vi "Solve_Special_PRB_101_Subtracks-3.vi"(3 "error IN":errorcluster, 5 "[IN] Subtracks":T1(array[cluster])) -> (0 "error OUT":errorcluster, 1 "[OUT] Special case!":bool, 2 "[OUT] Subtracks":T1(array[cluster]))   [LabVIEW 2013]
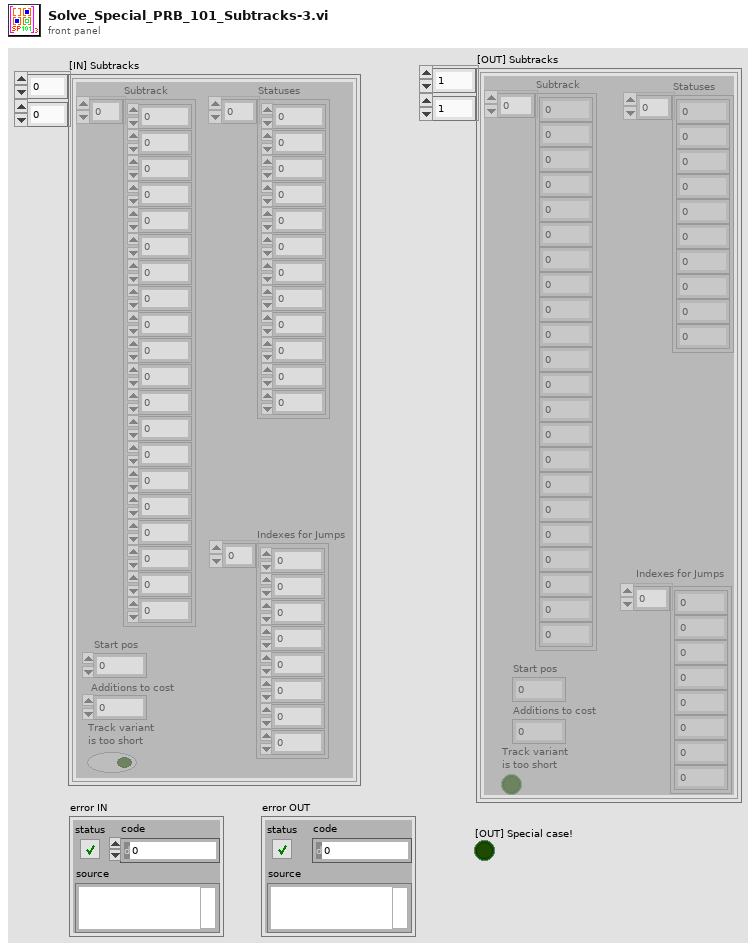
[diagram p1: front panel]
types:
  T1 = cluster{"Subtrack":dbl[], "Statuses":i16[], "Start pos":i32, "Additions to cost":i32, "Track variant \nis too short":bool, "Indexes for Jumps":i32[]}[][]
  T2 = cluster{"Subtrack":dbl[], "Statuses":i16[], "Start pos":i32, "Additions to cost":i32, "Track variant \nis too short":bool, "Indexes for Jumps":i32[]}
  T3 = cluster{"Subtrack":dbl[], "Statuses":i16[], "Start pos":i32, "Additions to cost":i32, "Track variant \nis too short":bool, "Indexes for Jumps":i32[]}[]
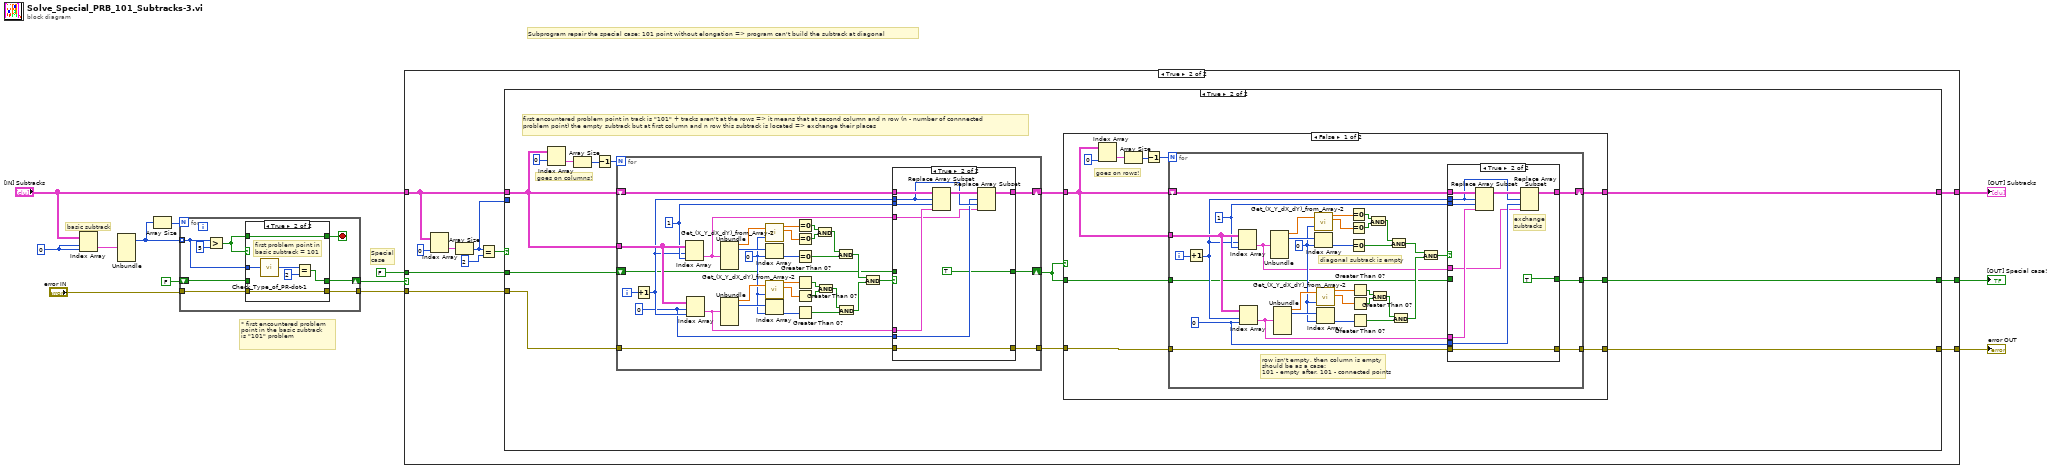
[diagram p0: block diagram]
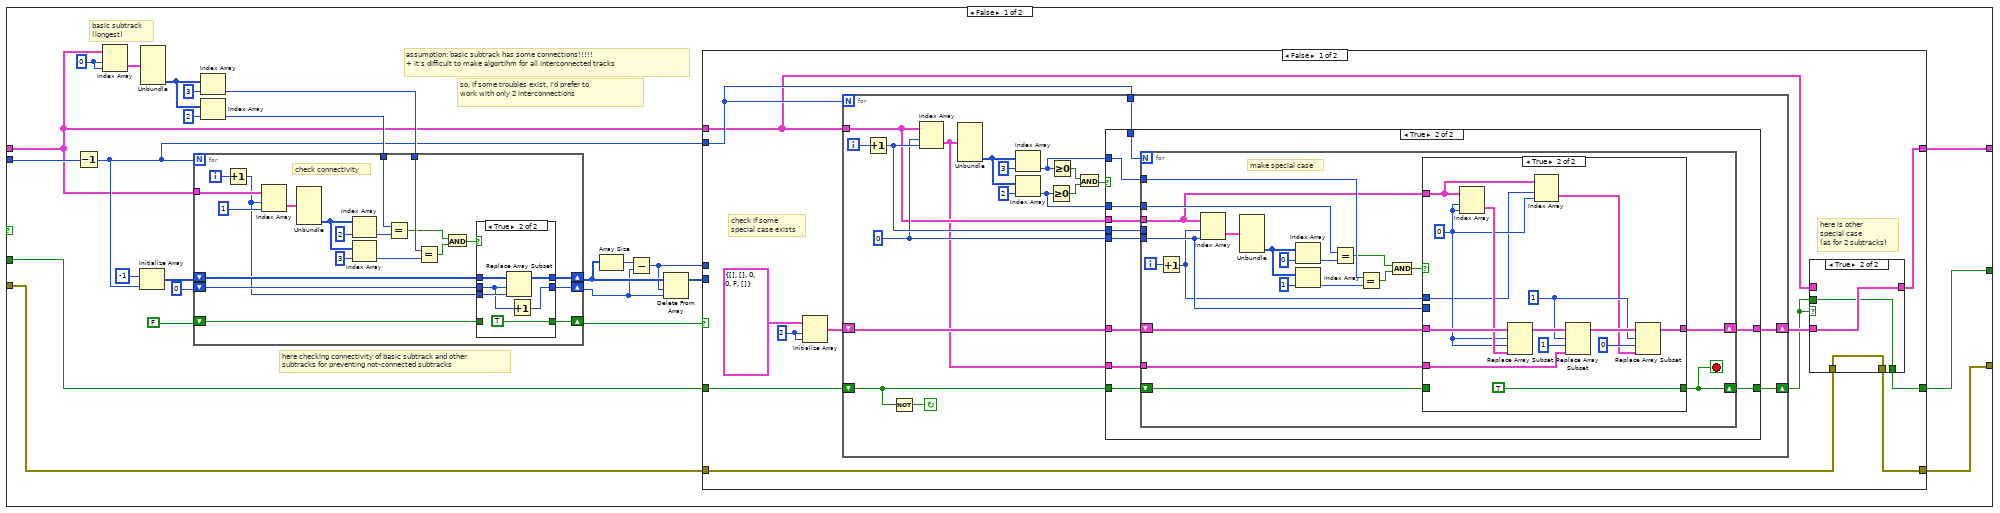
[diagram p3: hidden frame]
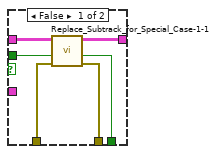
[diagram p4: hidden frame]
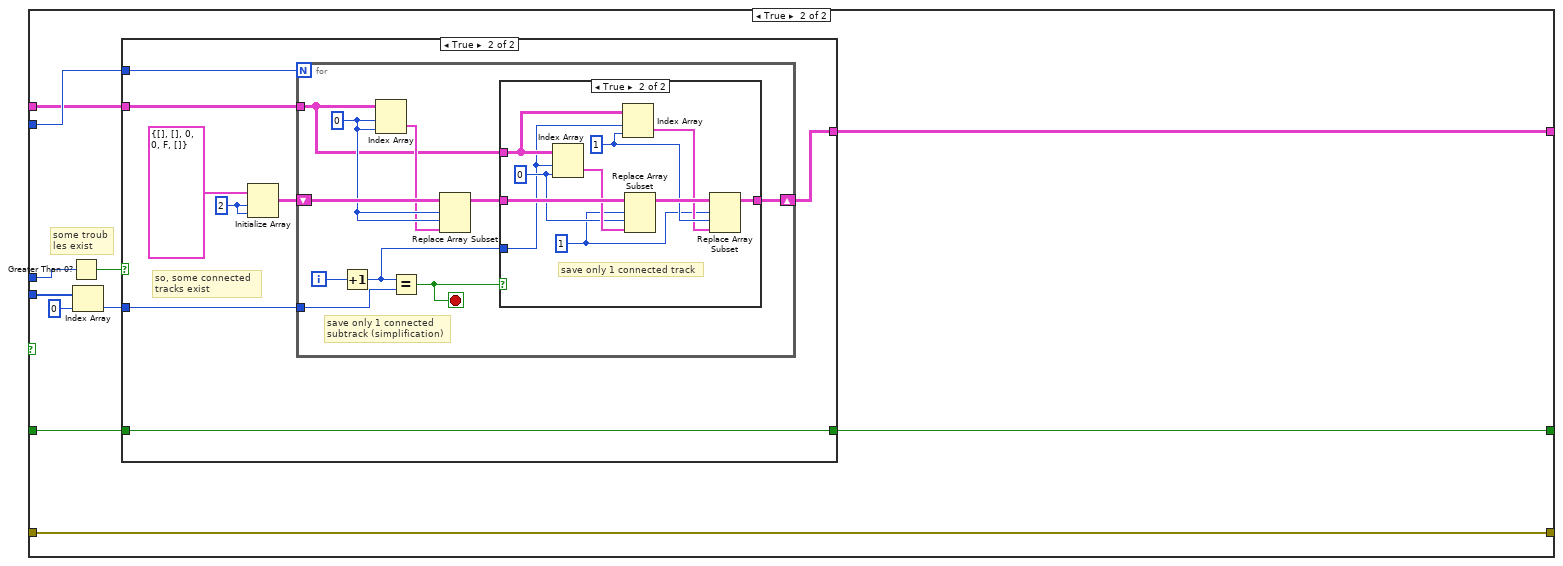
[diagram p7: hidden frame]
diagram:
  w13 = 0 ("index (row)")
  # "* first encountered problem\npoint in the basic subtrack\nis \"101\" problem"
  # "Special \ncase"
  # "Subprogram repair the special case: 101 point without elongation => program can't build the subtrack at diagonal"
  # "basic subtrack"
  n1 = Index Array(array="[IN] Subtracks", index (row)=w13, index (col)=w13) -> (element=w12:T2)
  n2 = Unbundle(w12) -> ("Statuses"=w10:i16[])  [unwired: 5 out]
  n3 = Array Size(array=w10) -> (size(s)=w11:i32)
  n4 = for {
    N: w11 -> [_]
    tunnel: w10 -> [w20] mode=indexing
    shift-right: [w16] -> w1
    shift-left: FALSE -> [w19]
    tunnel: "error IN" -> [w15]
    tunnel: [w14] -> w7
    stop <- w17 stop-if-true
    n5 = Greater?(x=w20, y=i16 5) -> (0:w18:bool)
    n6 = case shown="True" w18 {
      tunnel: w20 -> [_ w28]
      tunnel: w19 -> [w23 _]
      tunnel: w18 -> [w24 w27]
      tunnel: [w24 w27] -> w17
      tunnel: [w23 w26] -> w16
      tunnel: w15 -> [w22 w25]
      tunnel: [w22 w25] -> w14
      frame False {
      }
      frame True {
        # "first problem point in \nbasic subtrack = 101"
        n7 = call "Check_Type_of_PR-dot-1.vi"("[IN] dot status"=w28) -> ("[OUT] Type of\nproblem dot"=w30:i32)
        n8 = Equal?(x=w30, y=2) -> (x = y?=w26:bool)
      }
    }
  }
  n9 = case shown="True" w1 {
    tunnel: w7 -> [w31 w44]
    tunnel: "[IN] Subtracks" -> [w33 w39]
    tunnel: FALSE -> [w32 w43]
    tunnel: [w32 w42] -> w4
    tunnel: [w33 w41] -> w3
    tunnel: [w31 w40] -> w2
    frame False {
    }
    frame True {
      n10 = Index Array(array=w39, index (col)=0) -> (element=w37:T3)  [unwired: 1 in]
      n11 = Array Size(array=w37) -> (size(s)=w34:i32)
      n12 = Equal?(x=w34, y=2) -> (x = y?=w35:bool)
      n13 = case shown="True" w35 {
        tunnel: w44 -> [w48 w243]
        tunnel: w39 -> [w50 w242]
        tunnel: w43 -> [w68 w241]
        tunnel: [w46 w237] -> w42
        tunnel: [w45 w236] -> w41
        tunnel: [w47 w235] -> w40
        tunnel: w34 -> [w69 _]
        frame False {
          w67 = 0 ("index (row)")
          # "so, if some troubles exist, I'd prefer to \nwork with only 2 interconnections"
          # "assumption: basic subtrack has some connections!!!!!\n+ it's difficult to make algortihm for all interconnected tracks"
          # "here checking connectivity of basic subtrack and other \nsubtracks for preventing not-connected subtracks"
          # "basic subtrack \n(longest)"
          n14 = Decrement(x=w69) -> (x-1=w52:i32)
          n15 = Index Array(array=w50, index (row)=w67, index (col)=w67) -> (element=w66:T2)
          n16 = Initialize Array(-1, w52) -> (w59:i32[])
          n17 = Unbundle(w66) -> ("Indexes for Jumps"=w63:i32[])  [unwired: 5 out]
          n18 = Index Array(array=w63, index=3) -> (element=w60:i32)
          n19 = Index Array(array=w63, index=2) -> (element=w61:i32)
          n20 = for {
            N: w52 -> [_]
            tunnel: w61 -> [w213]
            tunnel: w60 -> [w211]
            shift-right: [w204] -> w56
            shift-left: w59 -> [w207]
            shift-right: [w201] -> w51
            shift-left: FALSE -> [w203]
            shift-right: [w202] -> w54
            shift-left: 0 -> [w206]
            tunnel: w50 -> [w221]
            i -> [w220]
            # "check connectivity"
            n21 = Increment(x=w220) -> (x+1=w205:i32)
            n22 = Index Array(array=w221, index (row)=w205, index (col)=1) -> (element=w216:T2)
            n23 = Unbundle(w216) -> ("Indexes for Jumps"=w215:i32[])  [unwired: 5 out]
            n24 = Index Array(array=w215, index=2) -> (element=w214:i32)
            n25 = Index Array(array=w215, index=3) -> (element=w212:i32)
            n26 = Equal?(x=w213, y=w214) -> (x = y?=w210:bool)
            n27 = Equal?(x=w211, y=w212) -> (x = y?=w209:bool)
            n28 = And(x=w210, y=w209) -> (x .and. y?=w208:bool)
            n29 = case shown="True" w208 {
              tunnel: w207 -> [w222 w230]
              tunnel: w206 -> [w223 w227]
              tunnel: w205 -> [_ w229]
              tunnel: [w222 w228] -> w204
              tunnel: w203 -> [w224 _]
              tunnel: [w223 w226] -> w202
              tunnel: [w224 TRUE] -> w201
              frame False {
              }
              frame True {
                n30 = Replace Array Subset(array=w230, new element=w229, index=w227) -> (w228:i32[])
                n31 = Increment(x=w227) -> (x+1=w226:i32)
              }
            }
          }
          n32 = Array Size(array=w56) -> (size(s)=w55:i32)
          n33 = Subtract(x=w55, y=w54) -> (x-y=w49:i32)
          n34 = Delete From Array(array=w56, length=w49, index=w54) -> (array with subset deleted=w53:i32[])  [unwired: 1 out]
          n35 = case shown="False" w51 {
            tunnel: w53 -> [_ w165]
            tunnel: w52 -> [w80 w169]
            tunnel: w50 -> [w74 w168]
            tunnel: w68 -> [w81 w162]
            tunnel: w49 -> [_ w167]
            tunnel: w48 -> [w73 w159]
            tunnel: [w72 w159] -> w47
            tunnel: [w75 w161] -> w45
            tunnel: [w70 w160] -> w46
            frame False {
              w78 = 2 ("dimension size")
              # "here is other \nspecial case\n(as for 2 subtracks)"
              # "check if some \nspecial case exists"
              n36 = Initialize Array(T2 {"Subtrack"=[], "Statuses"=[], "Start pos"=0, "Additions to cost"=0, "Track variant \nis too short"=FALSE, "Indexes for Jumps"=[]} ("element"), w78, w78) -> (w77:T1)
              n37 = for {
                N: w80 -> [_]
                shift-right: [w98] -> w71
                shift-left: w81 -> [w95]
                tunnel: w80 -> [w99]
                tunnel: w74 -> [w97]
                shift-right: [w94] -> w76
                shift-left: w77 -> [w96]
                i -> [w109]
                stop <- w93 continue-if-true
                w102 = 0 ("disabled index (col)")
                n38 = Increment(x=w109) -> (x+1=w103:i32)
                n39 = Not(x=w95) -> (.not. x?=w93:bool)
                n40 = Index Array(array=w97, index (row)=w102, index (col)=w103) -> (element=w91:T2)
                n41 = Unbundle(w91) -> ("Indexes for Jumps"=w106:i32[])  [unwired: 5 out]
                n42 = Index Array(array=w106, index=3) -> (element=w100:i32)
                n43 = Index Array(array=w106, index=2) -> (element=w101:i32)
                n44 = Greater Or Equal To 0?(x=w101) -> (x >= 0?=w104:bool)
                n45 = Greater Or Equal To 0?(x=w100) -> (x >= 0?=w105:bool)
                n46 = And(x=w105, y=w104) -> (x .and. y?=w92:bool)
                n47 = case shown="True" w92 {
                  tunnel: w97 -> [_ w122]
                  tunnel: w103 -> [_ w121]
                  tunnel: w102 -> [_ w120]
                  tunnel: w101 -> [_ w119]
                  tunnel: w100 -> [_ w118]
                  tunnel: w99 -> [_ w117]
                  tunnel: w95 -> [w110 w116]
                  tunnel: [w110 w115] -> w98
                  tunnel: w96 -> [w111 w114]
                  tunnel: [w111 w113] -> w94
                  tunnel: w91 -> [_ w112]
                  frame False {
                  }
                  frame True {
                    n48 = for {
                      N: w117 -> [_]
                      tunnel: w121 -> [_]
                      tunnel: w120 -> [w132]
                      tunnel: w119 -> [w138]
                      tunnel: w118 -> [w137]
                      shift-right: [w126] -> w115
                      shift-left: w116 -> [w131]
                      tunnel: w122 -> [w133]
                      shift-right: [w127] -> w113
                      shift-left: w114 -> [w129]
                      tunnel: w112 -> [w123]
                      i -> [w125]
                      stop <- w126 stop-if-true
                      # "make special case"
                      n49 = Increment(x=w125) -> (x+1=w124:i32)
                      n50 = Index Array(array=w133, index (row)=w124, index (col)=w132) -> (element=w128:T2)
                      n51 = Unbundle(w128) -> ("Indexes for Jumps"=w140:i32[])  [unwired: 5 out]
                      n52 = Index Array(array=w140, index=0) -> (element=w139:i32)
                      n53 = Index Array(array=w140, index=1) -> (element=w136:i32)
                      n54 = Equal?(x=w138, y=w139) -> (x = y?=w135:bool)
                      n55 = Equal?(x=w137, y=w136) -> (x = y?=w134:bool)
                      n56 = And(x=w135, y=w134) -> (x .and. y?=w130:bool)
                      n57 = case shown="True" w130 {
                        tunnel: w133 -> [_ w148]
                        tunnel: w124 -> [_ w147]
                        tunnel: w132 -> [_ _]
                        tunnel: w131 -> [w144 _]
                        tunnel: [w144 TRUE] -> w126
                        tunnel: w129 -> [w143 w157]
                        tunnel: w123 -> [_ w153]
                        tunnel: [w143 w150] -> w127
                        frame False {
                        }
                        frame True {
                          w146 = 1 ("disabled index (col)")
                          w149 = 0 ("index (row)")
                          n58 = Index Array(array=w148, index (row)=w149, index (col)=w149) -> (element=w156:T2)
                          n59 = Replace Array Subset(array=w157, new element=w156, index (row)=w149, index (col)=w149) -> (w155:T1)
                          n60 = Index Array(array=w148, index (row)=w147, index (col)=w149) -> (element=w145:T2)
                          n61 = Replace Array Subset(array=w155, new element=w153, index (row)=w146, index (col)=1 ("disabled index (col)")) -> (w152:T1)
                          n62 = Replace Array Subset(array=w152, new element=w145, index (row)=w146, index (col)=0 ("disabled index (col)")) -> (w150:T1)
                        }
                      }
                    }
                  }
                }
              }
              n63 = case shown="True" w71 {
                tunnel: w76 -> [_ w90]
                tunnel: [w82 w90] -> w75
                tunnel: w74 -> [w87 _]
                tunnel: w73 -> [w86 w89]
                tunnel: [w85 w89] -> w72
                tunnel: w71 -> [w84 w88]
                tunnel: [w83 w88] -> w70
                frame False {
                  n64 = call "Replace_Subtrack_for_Special_Case-1-1.vi"("error IN"=w86, "[IN] Special case?"=w84, "[IN] Subtracks"=w87) -> ("error OUT"=w85:errorcluster, "[OUT Special case?"=w83:bool, "[OUT] Subtracks"=w82:T1)  [unwired: 2 in]
                }
                frame True {
                }
              }
            }
            frame True {
              # "some troub\nles exist"
              n65 = Greater Than 0?(x=w167) -> (x > 0?=w166:bool)
              n66 = Index Array(array=w165, index=0) -> (element=w163:i32)
              n67 = case shown="True" w166 {
                tunnel: w169 -> [_ w179]
                tunnel: w168 -> [w171 w177]
                tunnel: w163 -> [_ w178]
                tunnel: w162 -> [w170 w173]
                tunnel: [w170 w173] -> w160
                tunnel: [w171 w172] -> w161
                frame False {
                  # "no troubles => save all subtracks"
                }
                frame True {
                  w175 = 2 ("dimension size")
                  # "so, some connected \ntracks exist"
                  n68 = Initialize Array(T2 {"Subtrack"=[], "Statuses"=[], "Start pos"=0, "Additions to cost"=0, "Track variant \nis too short"=FALSE, "Indexes for Jumps"=[]} ("element"), w175, w175) -> (w174:T1)
                  n69 = for {
                    N: w179 -> [_]
                    tunnel: w178 -> [w188]
                    tunnel: w177 -> [w182]
                    shift-right: [w181] -> w172
                    shift-left: w174 -> [w187]
                    i -> [w189]
                    stop <- w183 stop-if-true
                    w186 = 0 ("index (row)")
                    # "save only 1 connected \nsubtrack (simplification)"
                    n70 = Increment(x=w189) -> (x+1=w180:i32)
                    n71 = Index Array(array=w182, index (row)=w186, index (col)=w186) -> (element=w185:T2)
                    n72 = Equal?(x=w180, y=w188) -> (x = y?=w183:bool)
                    n73 = Replace Array Subset(array=w187, new element=w185, index (row)=w186, index (col)=w186) -> (w184:T1)
                    n74 = case shown="True" w183 {
                      tunnel: w184 -> [w190 w200]
                      tunnel: w182 -> [_ w197]
                      tunnel: [w190 w192] -> w181
                      tunnel: w180 -> [_ w195]
                      frame False {
                      }
                      frame True {
                        w191 = 1 ("disabled index (row)")
                        w194 = 1 ("disabled index (col)")
                        w198 = 0 ("index (row)")
                        # "save only 1 connected track"
                        n75 = Index Array(array=w197, index (row)=w195, index (col)=w198) -> (element=w199:T2)
                        n76 = Index Array(array=w197, index (row)=w195, index (col)=w194) -> (element=w193:T2)
                        n77 = Replace Array Subset(array=w200, new element=w199, index (row)=w191, index (col)=w198) -> (w196:T1)
                        n78 = Replace Array Subset(array=w196, new element=w193, index (row)=w191, index (col)=w194) -> (w192:T1)
                      }
                    }
                  }
                }
              }
            }
          }
        }
        frame True {
          # "goes on columns!"
          # "first encountered problem point in track is \"101\" + tracks aren't at the rows => it means that at second column and n row (n - number of connnected\nproblem point) the empty subtrack but at first column and n row this subtrack is located => exchange their places"
          n79 = Index Array(array=w242, index (row)=0 ("disabled index (col)")) -> (element=w234:T3)  [unwired: 1 in]
          n80 = Array Size(array=w234) -> (size(s)=w233:i32)
          n81 = Decrement(x=w233) -> (x-1=w232:i32)
          n82 = for {
            N: w232 -> [_]
            tunnel: w242 -> [w277]
            shift-right: [w248] -> w239
            shift-left: w242 -> [w254]
            tunnel: w243 -> [w247]
            tunnel: [w246] -> w238
            shift-right: [w244] -> w240
            shift-left: w241 -> [w245]
            i -> [w278]
            w262 = 0 ("index")
            w249 = 0 ("disabled index (col)")
            w251 = 1 ("disabled index (col)")
            n83 = Increment(x=w278) -> (x+1=w250:i32)
            n84 = Index Array(array=w277, index (row)=w250, index (col)=w251) -> (element=w253:T2)
            n85 = Index Array(array=w277, index (row)=w249, index (col)=w250) -> (element=w252:T2)
            n86 = Unbundle(w253) -> ("Subtrack"=w274:dbl[], "Statuses"=w276:i16[])  [unwired: 4 out]
            n87 = Unbundle(w252) -> ("Subtrack"=w273:dbl[], "Statuses"=w275:i16[])  [unwired: 4 out]
            n88 = call "Get_(X_Y_dX_dY)_from_Array-2.vi"("(X,Y,dX,dY)"=w274, "Index of Displacement"=w262) -> ("X"=w272:dbl, "Y"=w271:dbl)  [unwired: 2 out]
            n89 = Index Array(array=w276, index=w262) -> (element=w270:i16)
            n90 = call "Get_(X_Y_dX_dY)_from_Array-2.vi"("(X,Y,dX,dY)"=w273, "Index of Displacement"=w262) -> ("X"=w265:dbl, "Y"=w264:dbl)  [unwired: 2 out]
            n91 = Index Array(array=w275, index=w262) -> (element=w263:i16)
            n92 = Equal To 0?(x=w272) -> (x = 0?=w269:bool)
            n93 = Equal To 0?(x=w271) -> (x = 0?=w268:bool)
            n94 = Equal To 0?(x=w270) -> (x = 0?=w266:bool)
            n95 = Greater Than 0?(x=w265) -> (x > 0?=w261:bool)
            n96 = Greater Than 0?(x=w264) -> (x > 0?=w260:bool)
            n97 = Greater Than 0?(x=w263) -> (x > 0?=w258:bool)
            n98 = And(x=w269, y=w268) -> (x .and. y?=w267:bool)
            n99 = And(x=w261, y=w260) -> (x .and. y?=w259:bool)
            n100 = And(x=w267, y=w266) -> (x .and. y?=w257:bool)
            n101 = And(x=w259, y=w258) -> (x .and. y?=w256:bool)
            n102 = And(x=w257, y=w256) -> (x .and. y?=w255:bool)
            n103 = case shown="True" w255 {
              tunnel: w254 -> [w281 w291]
              tunnel: w253 -> [_ w285]
              tunnel: w252 -> [_ w289]
              tunnel: w250 -> [_ w287]
              tunnel: w251 -> [_ w290]
              tunnel: w249 -> [_ w286]
              tunnel: [w281 w284] -> w248
              tunnel: w247 -> [w280 w283]
              tunnel: [w280 w283] -> w246
              tunnel: w245 -> [w279 _]
              tunnel: [w279 TRUE] -> w244
              frame False {
              }
              frame True {
                n104 = Replace Array Subset(array=w291, new element=w289, index (row)=w287, index (col)=w290) -> (w288:T1)
                n105 = Replace Array Subset(array=w288, new element=w285, index (row)=w286, index (col)=w287) -> (w284:T1)
              }
            }
          }
          n106 = case shown="False" w240 {
            tunnel: w239 -> [w297 w352]
            tunnel: w238 -> [w295 w350]
            tunnel: w240 -> [w296 w351]
            tunnel: [w294 w352] -> w236
            tunnel: [w293 w351] -> w237
            tunnel: [w292 w350] -> w235
            frame False {
              # "goes on rows!"
              n107 = Index Array(array=w297, index (col)=0 ("index (row)")) -> (element=w300:T3)  [unwired: 1 in]
              n108 = Array Size(array=w300) -> (size(s)=w301:i32)
              n109 = Decrement(x=w301) -> (x-1=w299:i32)
              n110 = for {
                N: w299 -> [_]
                shift-right: [w305] -> w294
                shift-left: w297 -> [w312]
                tunnel: w297 -> [w326]
                tunnel: w296 -> [w304]
                tunnel: w295 -> [w310]
                tunnel: [w303] -> w293
                tunnel: [w302] -> w292
                i -> [w336]
                w307 = 0 ("disabled index (col)")
                w316 = 0 ("index")
                w309 = 1 ("disabled index (col)")
                # "row isn't empty, then column is empty\nshould be as a case:\n101 - empty after, 101 - connected points"
                # "diagonal subtrack is empty"
                n111 = Increment(x=w336) -> (x+1=w308:i32)
                n112 = Index Array(array=w326, index (row)=w308, index (col)=w309) -> (element=w306:T2)
                n113 = Index Array(array=w326, index (row)=w308, index (col)=w307) -> (element=w311:T2)
                n114 = Unbundle(w306) -> ("Subtrack"=w334:dbl[], "Statuses"=w335:i16[])  [unwired: 4 out]
                n115 = Unbundle(w311) -> ("Subtrack"=w324:dbl[], "Statuses"=w325:i16[])  [unwired: 4 out]
                n116 = call "Get_(X_Y_dX_dY)_from_Array-2.vi"("(X,Y,dX,dY)"=w334, "Index of Displacement"=w316) -> ("X"=w333:dbl, "Y"=w332:dbl)  [unwired: 2 out]
                n117 = Index Array(array=w335, index=w316) -> (element=w331:i16)
                n118 = call "Get_(X_Y_dX_dY)_from_Array-2.vi"("(X,Y,dX,dY)"=w324, "Index of Displacement"=w316) -> ("X"=w323:dbl, "Y"=w322:dbl)  [unwired: 2 out]
                n119 = Index Array(array=w325, index=w316) -> (element=w321:i16)
                n120 = Equal To 0?(x=w333) -> (x = 0?=w330:bool)
                n121 = Equal To 0?(x=w332) -> (x = 0?=w329:bool)
                n122 = Equal To 0?(x=w331) -> (x = 0?=w327:bool)
                n123 = Greater Than 0?(x=w323) -> (x > 0?=w320:bool)
                n124 = Greater Than 0?(x=w322) -> (x > 0?=w319:bool)
                n125 = Greater Than 0?(x=w321) -> (x > 0?=w317:bool)
                n126 = And(x=w330, y=w329) -> (x .and. y?=w328:bool)
                n127 = And(x=w320, y=w319) -> (x .and. y?=w318:bool)
                n128 = And(x=w328, y=w327) -> (x .and. y?=w315:bool)
                n129 = And(x=w318, y=w317) -> (x .and. y?=w314:bool)
                n130 = And(x=w315, y=w314) -> (x .and. y?=w313:bool)
                n131 = case shown="True" w313 {
                  tunnel: w312 -> [w338 w349]
                  tunnel: w311 -> [_ w347]
                  tunnel: w310 -> [w339 w341]
                  tunnel: w309 -> [_ w348]
                  tunnel: w308 -> [_ w344]
                  tunnel: w307 -> [_ w345]
                  tunnel: w306 -> [_ w343]
                  tunnel: [w338 w342] -> w305
                  tunnel: [w339 w341] -> w302
                  tunnel: w304 -> [w337 _]
                  tunnel: [w337 TRUE] -> w303
                  frame False {
                  }
                  frame True {
                    # "exchange \nsubtracks"
                    n132 = Replace Array Subset(array=w349, new element=w347, index (row)=w344, index (col)=w348) -> (w346:T1)
                    n133 = Replace Array Subset(array=w346, new element=w343, index (row)=w344, index (col)=w345) -> (w342:T1)
                  }
                }
              }
            }
            frame True {
            }
          }
        }
      }
    }
  }
  "error OUT" <- w2
  "[OUT] Subtracks" <- w3
  "[OUT] Special case!" <- w4
